vi "Register Logger.vi"(8 "error in (no error)":errorcluster, 10 "Logger Registration":T1, 11 "Log Manager Module in":refnum<class "Log Manager Module.lvclass">) -> (0 "error out":errorcluster, 3 "Log Manager Module out":refnum<class "Log Manager Module.lvclass">)   [LabVIEW 2020, in "VolatusData.lvlib" / "Log Manager Module.lvclass"]
uses:
  Log Manager Module.lvclass
  C:/dev/lv20CE/relink/lv-volatus/Volatus/Module/Module.lvclass
  Register Logger.ctl
  Volatus/MessageQ/MessageQ.lvclass
  Log Manager Module.lvclass/Log Manager Module.ctl
  Logger.ctl
  Logger State.ctl
  <vilib>/Utility/miscctls.llb/LVMapReplaceAction.ctl
  Volatus/Module/Module.lvclass/Module.ctl
  Volatus/Event Level.ctl
  Volatus/Module/Module.lvclass
  Volatus/Volatus.lvlib
  VolatusData.lvlib
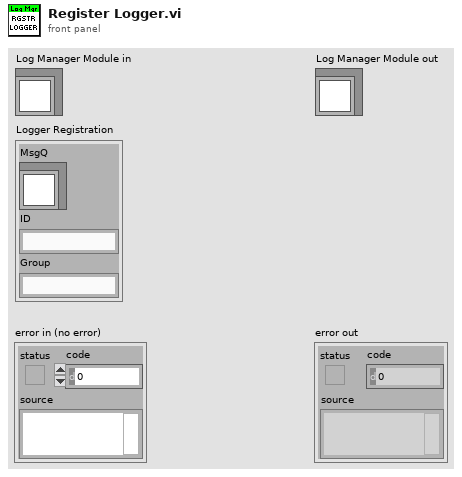
[diagram p1: front panel]
types:
  T1 = typedef "VolatusData.lvlib/Register Logger.ctl" = cluster{"MsgQ":refnum<class "MessageQ.lvclass">, "ID":string, "Group":string}
  T2 = typedef "LVMapReplaceAction.ctl" = enum32{"Modify Entry only if found", "Add or Modify Entry", "Delete Entry"}
  T3 = typedef "VolatusData.lvlib/Logger State.ctl" = enum16{"Unknown", "Idle", "Preparing", "Ready", "Logging", "Stopping"}
  T4 = typedef "VolatusData.lvlib/Log Manager Module.lvclass/Logger.ctl" = cluster{"ID":string, "MsgQ":refnum<class "MessageQ.lvclass">, "State":T3, "Group":string}
  T5 = typedef "VolatusData.lvlib/Log Manager Module.lvclass/Group Info.ctl" = cluster{"Name":string, "Loggers":map{string, T4}}
  T6 = typedef "Volatus.lvlib/Event Level.ctl" = enum16{"Debug", "Info", "Warning", "Error"}
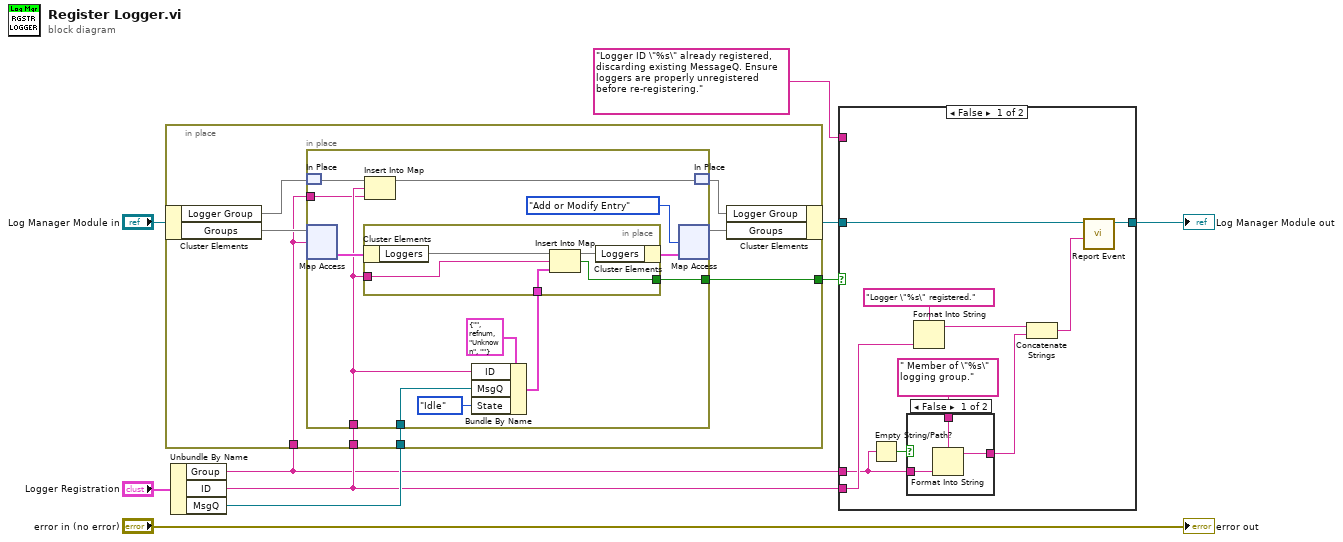
[diagram p0: block diagram]
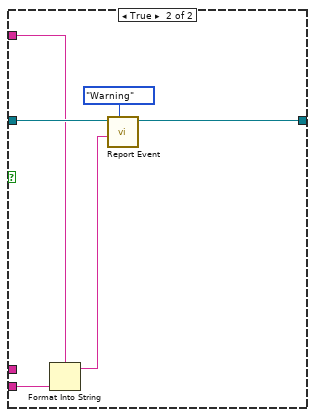
[diagram p3: hidden frame]
diagram:
  n1 = Unbundle By Name("Logger Registration") -> ("Group"=w1:string, "ID"=w3:string, "MsgQ"=w6:refnum<class "MessageQ.lvclass">)
  n2 = in-place {
    in-place-border: w3 -> [w18]
    in-place-border: w6 -> [w17]
    in-place-border: w1 -> [w11]
    in-place-border: [w15] -> w2
    n3 = in-place-cluster #1("Log Manager Module in") -> ("Logger Group"=w13:map{string, string}, "Groups"=w16:map{string, T5})
    n4 = in-place {
      in-place-border: w18 -> [w21]
      in-place-border: w17 -> [w29]
      in-place-border: [w24] -> w15
      in-place-border: w11 -> [w20]
      n5 = in-place-match #2(w13) -> (w23:map{string, string})
      n6 = in-place-map #3(w16, w11) -> (w27:T5)  [unwired: 1 in, 1 out]
      n7 = Insert Into Map(map in=w23, key=w21, value=w20) -> (map out=w22:map{string, string})  [unwired: 2 out]
      n8 = Bundle By Name(cluster=T4 {"ID"="", "MsgQ"=refnum, "State"=enum."Unknown", "Group"=""} ("value"), "ID"=w21, "MsgQ"=w29, "State"=Logger_State."Idle") -> (w25:T4)
      n9 = in-place {
        in-place-border: w25 -> [w33]
        in-place-border: w21 -> [w32]
        in-place-border: [w31] -> w24
        n10 = in-place-cluster #4(w27) -> ("Loggers"=w35:map{string, T4})
        n11 = Insert Into Map(map in=w35, key=w32, value=w33) -> (map out=w34:map{string, T4}, key already included?=w31:bool)  [unwired: 1 out]
        n12 = in-place-cluster #4("Loggers"=w34) -> (w26:T5)
      }
      n13 = in-place-map #3(w26, LVMapReplaceAction."Add or Modify Entry" ("action")) -> (w14:map{string, T5})  [unwired: 2 out]
      n14 = in-place-match #2(w22) -> (w12:map{string, string})
    }
    n15 = in-place-cluster #1("Logger Group"=w12, "Groups"=w14) -> (w8:refnum<class "Log Manager Module.lvclass">)
  }
  n16 = case shown="False" w2 {
    tunnel: w8 -> [w45 w54]
    tunnel: [w44 w53] -> w5
    tunnel: "Logger ID \"%s\" already registered, discarding existing MessageQ. Ensure loggers are properly unregistered before re-registering." -> [_ w51]
    tunnel: w3 -> [w41 w50]
    tunnel: w1 -> [w39 _]
    frame False {
      n17 = Empty String/Path?(string/path=w39) -> (empty?=w40:bool)
      n18 = case shown="False" w40 {
        tunnel: w39 -> [w48 _]
        tunnel: " Member of \"%s\" logging group." -> [w47 _]
        tunnel: [w46 _] -> w36
        frame False {
          n19 = Format Into String(format string=w47, w48) -> (resulting string=w46:string)  [unwired: 2 in, 1 out]
        }
        frame True {
        }
      }
      n20 = Format Into String(format string="Logger \"%s\" registered.", w41) -> (resulting string=w42:string)  [unwired: 2 in, 1 out]
      n21 = Concatenate Strings(w42, w36) -> (w37:string)
      n22 = call "Report Event.vi"("Message"=w37, "Module in"=w45) -> ("Module out"=w44:refnum<class "Log Manager Module.lvclass">)  [unwired: 8 in, 1 out]
    }
    frame True {
      n23 = Format Into String(format string=w51, w50) -> (resulting string=w49:string)  [unwired: 2 in, 1 out]
      n24 = call "Report Event.vi"("Level (Info)"=Event_Level."Warning", "Message"=w49, "Module in"=w54) -> ("Module out"=w53:refnum<class "Log Manager Module.lvclass">)  [unwired: 7 in, 1 out]
    }
  }
  "Log Manager Module out" <- w5
  "error out" <- "error in (no error)"
